vi "Save Settings.vi"(8 "error in (no error)":errorcluster) -> (0 "error out":errorcluster)   [LabVIEW 2013]
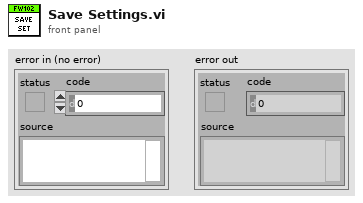
[diagram p1: front panel]
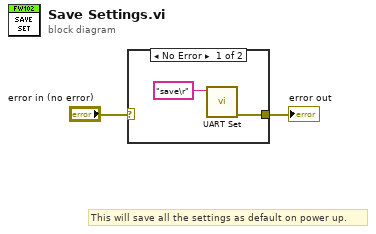
[diagram p0: block diagram]
diagram:
  # "This will save all the settings as default on power up."
  n1 = case shown="No Error" "error in (no error)" {
    selector: "error in (no error)" -> [_ w5]
    tunnel: [w4 w5] -> w2
    frame No Error {
      n2 = call "UART Set.vi"("Command"="save\r" ("Input Command String")) -> ("error out"=w4:errorcluster)  [unwired: 10 in]
    }
    frame Error {
    }
  }
  "error out" <- w2
